vi "REACTOR__SET_PARAMETROS_MEDIDA.vi"(6 "error in (no error)":errorcluster, 7 "Index":i8) -> (0 "error out":errorcluster, 2 "resulting string 1":string="Mide Bronkhorst 1, mide Alicats 1,  y pausa 1.0s", 3 "Cancelled?":bool)   [LabVIEW 2017]
doc: "Use this template to create a dialog box. This template polls the state of the buttons on the front panel and does not use events. Use the Dialog Using Events template (not available in Base package) to create a dialog box with event handling."
panel:
  in  "Mide Alicats":bool=TRUE
  in  "Mide Temperaturas":bool=TRUE
  in  "Muestreo (s)":dbl=0.1 format="%.1f"
  in  "Cancel":bool
  in  "OK":bool
  # "MEDIR PARAMETROS"
  # "Noviembre 2022 V1.0  a-sslcdms"
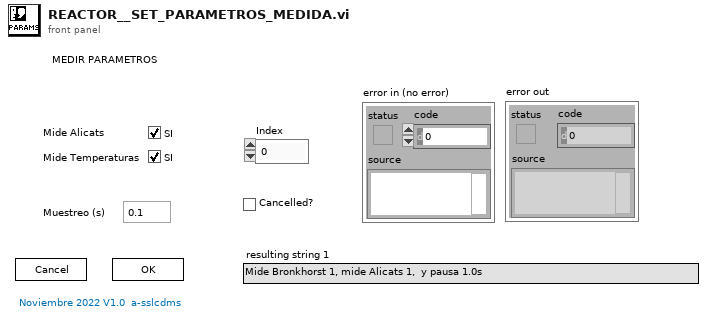
[diagram p1: front panel]
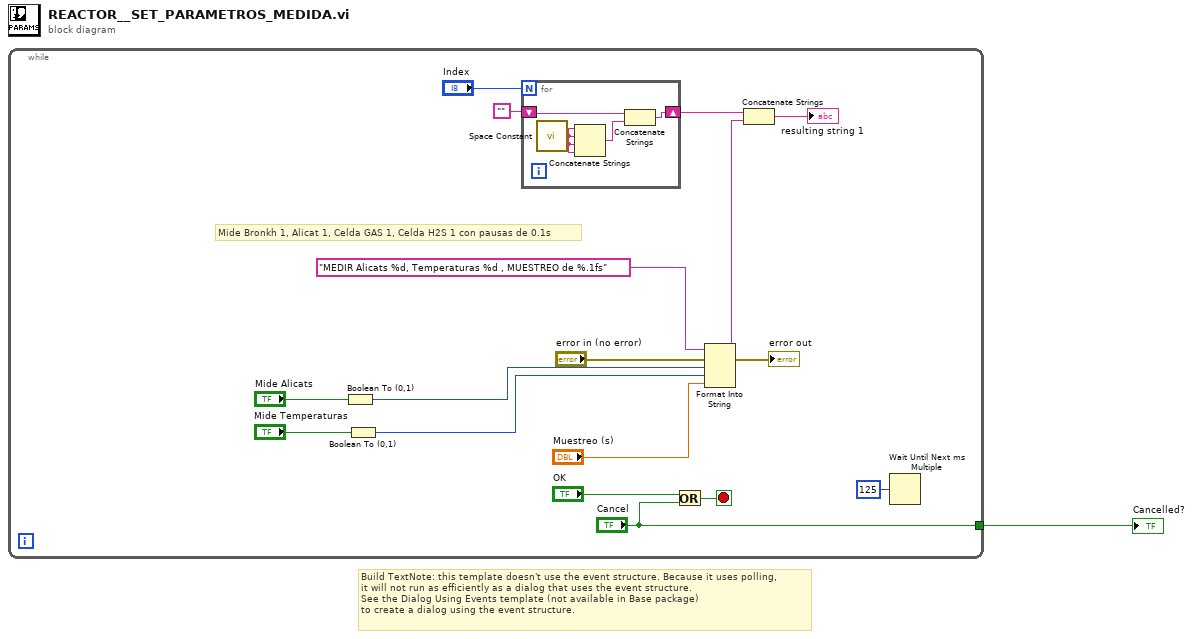
[diagram p0: block diagram]
diagram:
  # "Build TextNote: this template doesn't use the event structure. Because it uses polling, \nit will not run as efficiently as a dialog that uses the event structure.\nSee the Dialog Using Events template (not available in Base package) \nto create a dialog using the event structure."
  n1 = while {
    tunnel: ["Cancel"] -> w1
    stop <- w17 stop-if-true
    # "Mide Bronkh 1, Alicat 1, Celda GAS 1, Celda H2S 1 con pausas de 0.1s"
    n2 = Boolean To (0,1)(Boolean="Mide Alicats") -> (0, 1=w6:i16)
    n3 = Boolean To (0,1)(Boolean="Mide Temperaturas") -> (0, 1=w5:i16)
    n4 = for {
      N: "Index" -> [_]
      shift-right: [w21] -> w9
      shift-left: "" -> [w20]
      n5 = call <vilib>:"Space Constant.vi"() -> ("String"=w19:string)
      n6 = Concatenate Strings(w19, w19, w19, w19) -> (w22:string)
      n7 = Concatenate Strings(w20, w22) -> (w21:string)
    }
    n8 = Or(x="OK", y="Cancel") -> (x .or. y?=w17:bool)
    n9 = Format Into String(format string="MEDIR Alicats %d, Temperaturas %d , MUESTREO de %.1fs", error in="error in (no error)", w6, w5, "Muestreo (s)") -> (resulting string=w7:string, error out=→"error out":errorcluster)  [unwired: 1 in]
    n10 = Concatenate Strings(w9, w7) -> (→"resulting string 1":string)
    n11 = Wait Until Next ms Multiple(millisecond multiple=u32 125) -> ()  [unwired: 1 out]
  }
  "Cancelled?" <- w1
